vi "Divide Term By Term Ved3d.vi"(8 "error in":errorcluster, 10 "Vec3d in 2":refnum<class "Vec3d Class.lvclass">, 11 "Vec3d in 1":refnum<class "Vec3d Class.lvclass">) -> (0 "error out":errorcluster, 3 "Vec3d Class out":refnum<class "Vec3d Class.lvclass">)   [LabVIEW 2011, in "Vec3d Class.lvclass"]
uses:
  Vec3d Class.lvclass
  Vec3d Class.lvclass/Vec3d Class.ctl
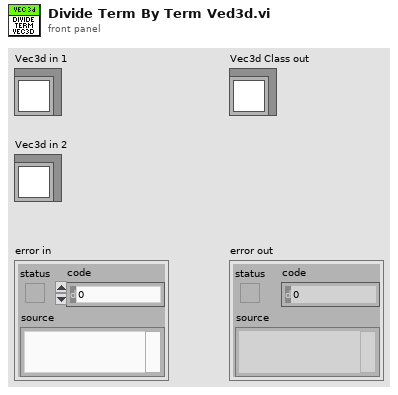
[diagram p1: front panel]
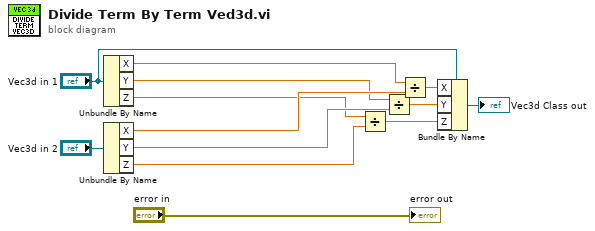
[diagram p0: block diagram]
diagram:
  n1 = Unbundle By Name("Vec3d in 1") -> ("X"=w12:dbl, "Y"=w10:dbl, "Z"=w8:dbl)
  n2 = Unbundle By Name("Vec3d in 2") -> ("X"=w11:dbl, "Y"=w9:dbl, "Z"=w7:dbl)
  n3 = Divide(x=w8, y=w7) -> (x/y=w3:dbl)
  n4 = Divide(x=w10, y=w9) -> (x/y=w4:dbl)
  n5 = Divide(x=w12, y=w11) -> (x/y=w5:dbl)
  n6 = Bundle By Name(cluster="Vec3d in 1", "X"=w5, "Y"=w4, "Z"=w3) -> (→"Vec3d Class out":refnum<class "Vec3d Class.lvclass">)
  "error out" <- "error in"
